vi "AddServerErrors.vi"(10 "Numeric":i32, 11 "Numeric 2":i32) -> (3 "Cmd Log":T1(array[cluster]))   [LabVIEW 2012]
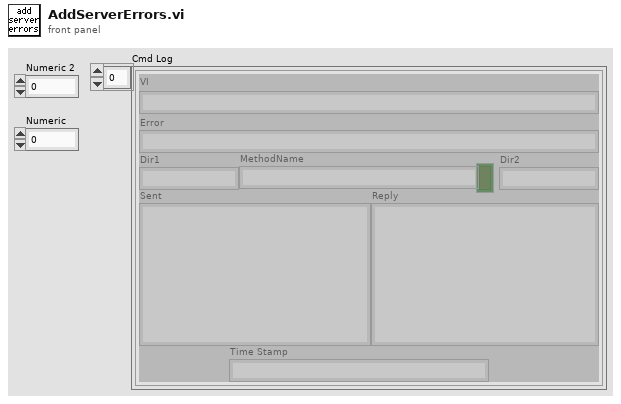
[diagram p1: front panel]
types:
  T1 = cluster{"Sent":string, "Reply":string, "MethodName":string, "success":bool, "Dir1":string, "Dir2":string, "Time Stamp":string, "Error":string, "VI":string}[]
  T2 = cluster{"Sent":string, "Reply":string, "MethodName":string, "success":bool, "Dir1":string, "Dir2":string, "Time Stamp":string, "Error":string, "VI":string}
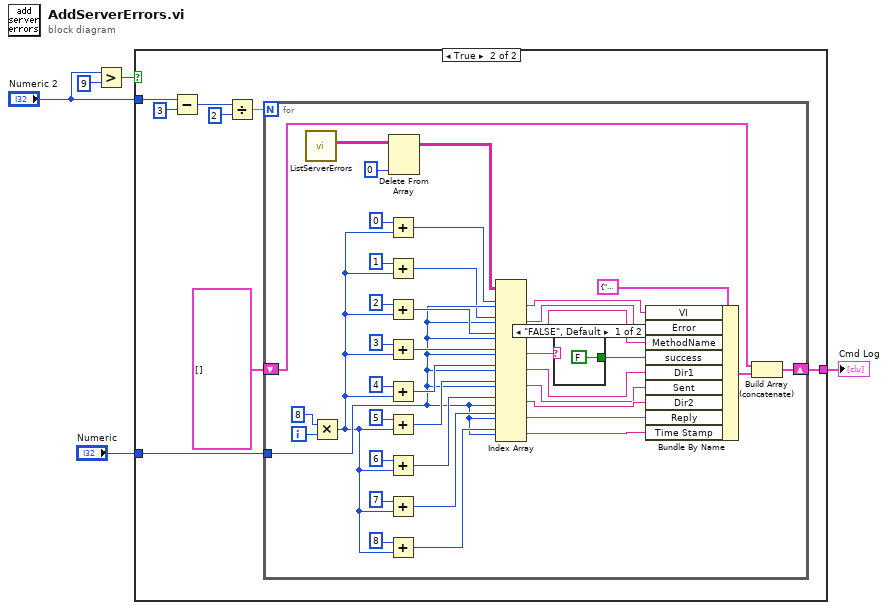
[diagram p0: block diagram]
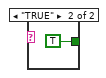
[diagram p3: hidden frame]
diagram:
  n1 = Greater?(x="Numeric 2", y=9) -> (0:w2:bool)
  n2 = case shown="True" w2 {
    tunnel: "Numeric 2" -> [_ w13]
    tunnel: [_ w8] -> w1
    tunnel: "Numeric" -> [_ w7]
    frame False {
    }
    frame True {
      n3 = Subtract(x=w13, y=3) -> (x-y=w11:i32)
      n4 = Divide(x=w11, y=2) -> (x/y=w9:dbl)
      n5 = for {
        N: w9 -> [_]
        shift-right: [w51] -> w8
        shift-left: T1 [] ("Cmd Log") -> [w50]
        tunnel: w7 -> [w18]
        i -> [w44]
        n6 = call <userlib>:"ListServerErrors.vi"() -> ("Array"=w45:string[][])  [unwired: 10 in, 1 out]
        n7 = Multiply(x=8, y=w44) -> (x*y=w15:i32)
        n8 = Add(x=0, y=w15) -> (x+y=w16:i32)
        n9 = Add(x=1, y=w15) -> (x+y=w17:i32)
        n10 = Add(x=2, y=w15) -> (x+y=w42:i32)
        n11 = Add(x=3, y=w15) -> (x+y=w41:i32)
        n12 = Add(x=4, y=w15) -> (x+y=w40:i32)
        n13 = Add(x=5, y=w15) -> (x+y=w39:i32)
        n14 = Add(x=6, y=w15) -> (x+y=w38:i32)
        n15 = Add(x=7, y=w15) -> (x+y=w37:i32)
        n16 = Add(x=8, y=w15) -> (x+y=w36:i32)
        n17 = Delete From Array(array=w45, index (col)=0 ("disabled index (col)")) -> (array with subset deleted=w46:string[][])  [unwired: 2 in, 1 out]
        n18 = Index Array(array=w46, index (row) #1=w16, index (col) #1=w18, index (row) #2=w17, index (col) #2=w18, index (row) #3=w42, index (col) #3=w18, index (row) #4=w41, index (col) #4=w18, index (row) #5=w40, index (col) #5=w18, index (row) #6=w39, index (col) #6=w18, index (row) #7=w38, index (col) #7=w18, index (row) #8=w37, index (col) #8=w18, index (row) #9=w36, index (col) #9=w18) -> (element #1=w19:string, element #2=w49:string, element #3=w48:string, element #4=w22:string, element #5=w23:string, element #6=w24:string, element #7=w25:string, element #8=w26:string, element #9=w27:string)
        n19 = case shown="\"FALSE\", Default" w22 {
          tunnel: [FALSE TRUE] -> w21
          frame "FALSE", Default {
          }
          frame "TRUE" {
          }
        }
        n20 = Bundle By Name(cluster=T2 {"Sent"="", "Reply"="", "MethodName"="", "success"=FALSE, "Dir1"="", "Dir2"="", "Time Stamp"="", "Error"="", "VI"=""} ("Log"), "VI"=w19, "Error"=w49, "MethodName"=w48, "success"=w21, "Dir1"=w23, "Sent"=w24, "Dir2"=w25, "Reply"=w26, "Time Stamp"=w27) -> (w52:T2)
        n21 = Build Array (concatenate)(w50, w52) -> (w51:T1)
      }
    }
  }
  "Cmd Log" <- w1
